vi "Read Packet Type.vi"(11 "ControlPacket in":refnum<class "ControlPacket.lvclass">) -> (2 "Control Packet Type":T1, 3 "ControlPacket out":refnum<class "ControlPacket.lvclass">)   [LabVIEW 2013, in "ControlPacket.lvclass"]
uses:
  ControlPacket.lvclass
  Control Packet Type -- enum.ctl
  ControlPacket.lvclass/ControlPacket.ctl
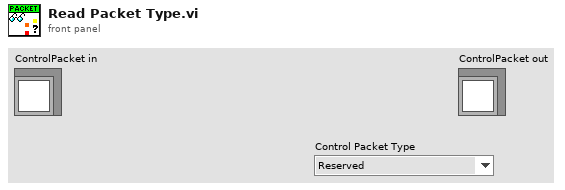
[diagram p1: front panel]
types:
  T1 = typedef "ControlPacket.lvclass/Control Packet Type -- enum.ctl" = enum16{"Reserved", "CONNECT", "CONNACK", "PUBLISH", "PUBACK", "PUBREC", "PUBREL", "PUBCOMP", "SUBSCRIBE", "SUBACK", "UNSUBSCRIBE", "UNSUBACK", "PINGREQ", "PINGRESP", "DISCONNECT", "Reserved(15)"}
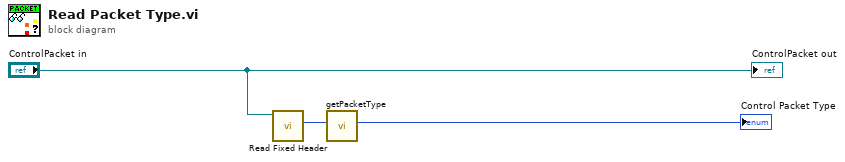
[diagram p0: block diagram]
diagram:
  n1 = call "Read Fixed Header.vi"("ControlPacket in"="ControlPacket in") -> ("Fixed Header"=w1:u8)  [unwired: 9 in, 1 out]
  n2 = call "getPacketType.vi"("Packet First Byte"=w1) -> ("Control Packet Type"=→"Control Packet Type":T1)  [unwired: 10 in]
  "ControlPacket out" <- "ControlPacket in"
